vi "1Lab.vi"() -> ()   [LabVIEW 2020]
panel:
  out "площадь треугольника":dbl
  out "периметр":dbl
  out "3 медиана":dbl
  out "2 медиана":dbl
  out "1 медиана":dbl
  in  "?":bool
  in  "3 сторона":dbl
  in  "2 сторона":dbl
  in  "1 сторона":dbl
  # "Рассчитывает площадь треуголинка через две формулы:\n1) через периметр\n3) через три медианы"
  # "считать через периметр"
  # "считать через медианы"
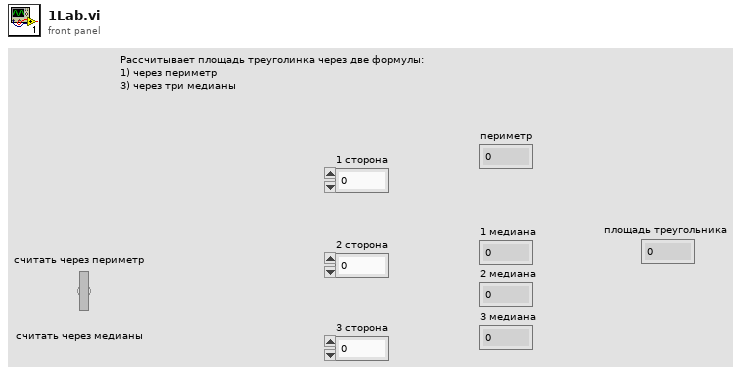
[diagram p1: front panel]
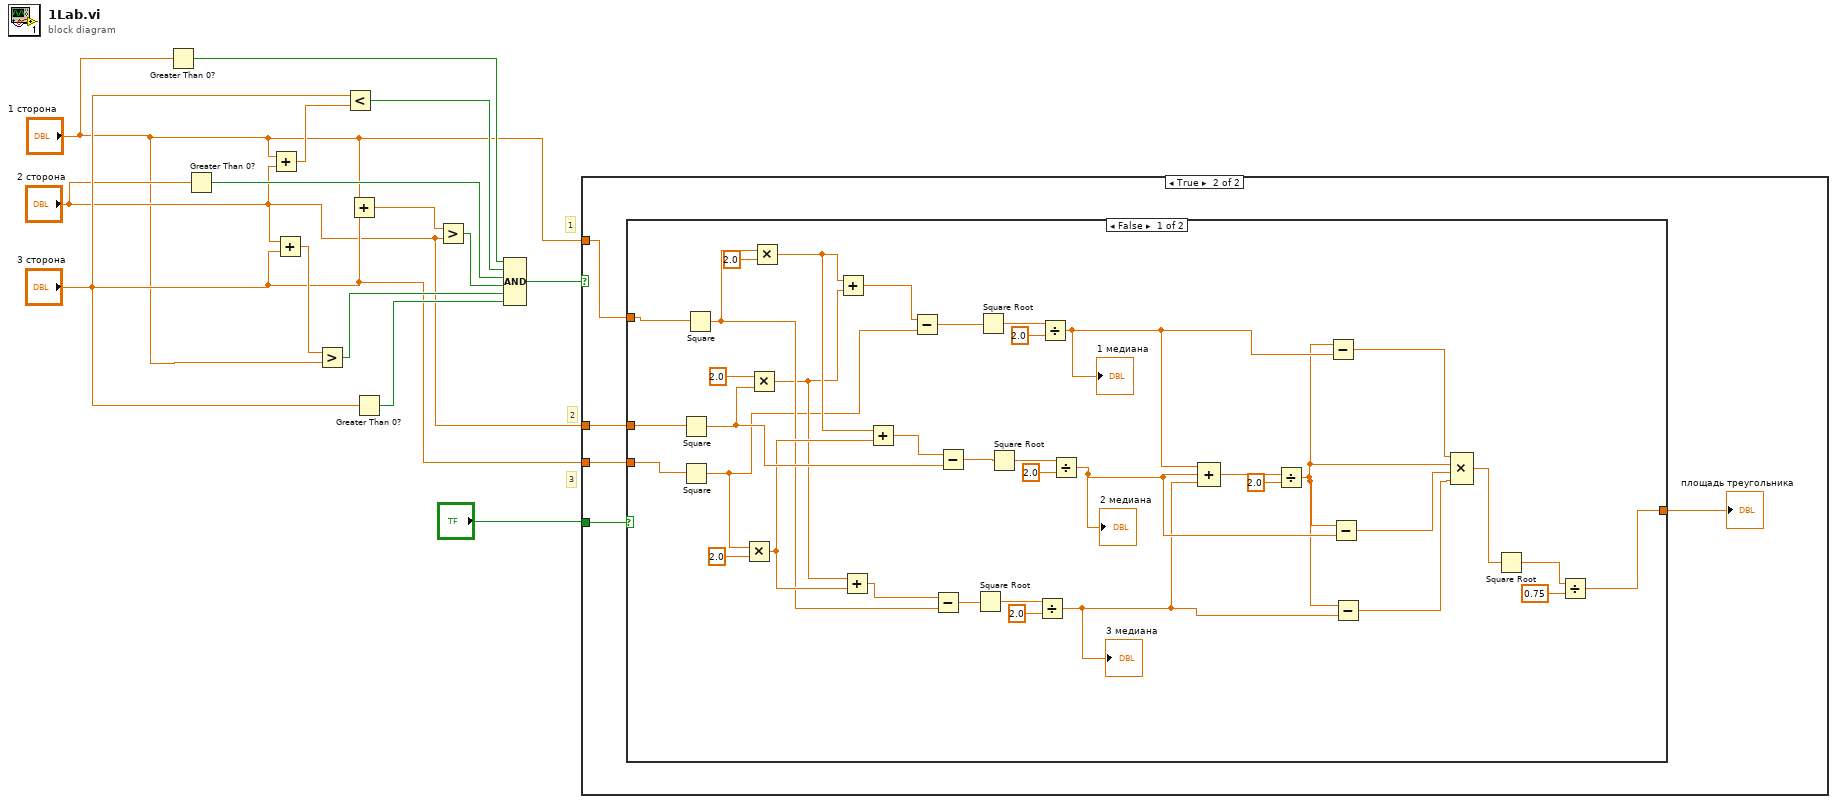
[diagram p0: block diagram]
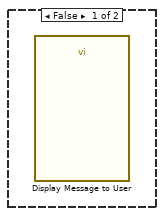
[diagram p2: hidden frame]
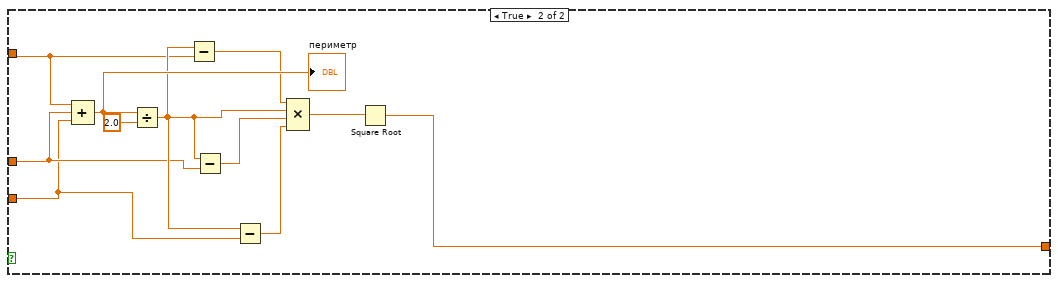
[diagram p3: hidden frame]
diagram:
  # "1"
  # "3"
  # "2"
  n1 = Greater Than 0?(x="1 сторона") -> (x > 0?=w11:bool)
  n2 = Greater Than 0?(x="2 сторона") -> (x > 0?=w9:bool)
  n3 = Add(x="1 сторона", y="2 сторона") -> (x+y=w14:dbl)
  n4 = Add(x="2 сторона", y="3 сторона") -> (x+y=w13:dbl)
  n5 = Greater?(x=w13, y="1 сторона") -> (0:w7:bool)
  n6 = Less?(x="3 сторона", y=w14) -> (x < y?=w10:bool)
  n7 = Add(x="1 сторона", y="3 сторона") -> (x+y=w12:dbl)
  n8 = Greater Than 0?(x="3 сторона") -> (x > 0?=w6:bool)
  n9 = Greater?(x=w12, y="2 сторона") -> (0:w8:bool)
  n10 = Compound Arithmetic op=AND(w11, w10, w9, w8, w7, w6) -> (w2:bool)
  n11 = case shown="True" w2 {
    tunnel: "1 сторона" -> [_ w16]
    tunnel: "2 сторона" -> [_ w18]
    tunnel: "3 сторона" -> [_ w17]
    tunnel: "?" -> [_ w19]
    frame False {
      n12 = call "Display Message to User"() -> ()  [unwired: 10 in, 2 out]
    }
    frame True {
      n13 = case shown="False" w19 {
        tunnel: w18 -> [w34 w59]
        tunnel: w17 -> [w33 w58]
        tunnel: w16 -> [w35 w60]
        tunnel: [w20 w57] -> w15
        frame False {
          n14 = Square(x=w34) -> (x^2=w54:dbl)
          n15 = Square(x=w33) -> (x^2=w43:dbl)
          n16 = Square(x=w35) -> (x^2=w48:dbl)
          n17 = Multiply(x=w43, y=2.0) -> (x*y=w52:dbl)
          n18 = Multiply(x=2.0, y=w54) -> (x*y=w46:dbl)
          n19 = Multiply(x=w48, y=2.0) -> (x*y=w51:dbl)
          n20 = Add(x=w51, y=w46) -> (x+y=w42:dbl)
          n21 = Add(x=w46, y=w52) -> (x+y=w47:dbl)
          n22 = Add(x=w51, y=w52) -> (x+y=w53:dbl)
          n23 = Subtract(x=w42, y=w43) -> (x-y=w44:dbl)
          n24 = Subtract(x=w47, y=w48) -> (x-y=w50:dbl)
          n25 = Subtract(x=w53, y=w54) -> (x-y=w56:dbl)
          n26 = Square Root(x=w50) -> (sqrt(x)=w49:dbl)
          n27 = Square Root(x=w44) -> (sqrt(x)=w45:dbl)
          n28 = Square Root(x=w56) -> (sqrt(x)=w55:dbl)
          n29 = Divide(x=w49, y=2.0) -> (x/y=w28:dbl)
          "3 медиана" <- w28
          n30 = Divide(x=w45, y=2.0) -> (x/y=w30:dbl)
          "1 медиана" <- w30
          n31 = Divide(x=w55, y=2.0) -> (x/y=w29:dbl)
          "2 медиана" <- w29
          n32 = Compound Arithmetic op=ADD(w30, w29, w28) -> (w32:dbl)
          n33 = Divide(x=w32, y=2.0) -> (x/y=w26:dbl)
          n34 = Subtract(x=w26, y=w30) -> (x-y=w27:dbl)
          n35 = Subtract(x=w26, y=w29) -> (x-y=w25:dbl)
          n36 = Subtract(x=w26, y=w28) -> (x-y=w24:dbl)
          n37 = Compound Arithmetic op=MULTIPLY(w27, w26, w25, w24) -> (w23:dbl)
          n38 = Square Root(x=w23) -> (sqrt(x)=w22:dbl)
          n39 = Divide(x=w22, y=0.75) -> (x/y=w20:dbl)
        }
        frame True {
          n40 = Compound Arithmetic op=ADD(w60, w59, w58) -> (w67:dbl)
          "периметр" <- w67
          n41 = Divide(x=w67, y=2.0) -> (x/y=w64:dbl)
          n42 = Subtract(x=w64, y=w60) -> (x-y=w65:dbl)
          n43 = Subtract(x=w64, y=w59) -> (x-y=w63:dbl)
          n44 = Subtract(x=w64, y=w58) -> (x-y=w62:dbl)
          n45 = Compound Arithmetic op=MULTIPLY(w65, w64, w63, w62) -> (w66:dbl)
          n46 = Square Root(x=w66) -> (sqrt(x)=w57:dbl)
        }
      }
      "площадь треугольника" <- w15
    }
  }
